vi "DoNanoCmd.vi"(4 "Relay Control Port":u32, 5 "Sense Resistor":dbl, 6 "Current Limit":dbl, 7 "Pin 2":u32, 8 "error in (no error)":errorcluster, 9 "Pin 1":u32, 10 "Nano Op":T1=enum."Get analog pin voltage", 11 "VISA resource name":refnum<visa-resource-name>="COM21") -> (0 "error out":errorcluster={"status"=FALSE, "code"=1073676294, "source"="VISA Read in DoNanoCmd.vi"}, 1 "Response length":i32, 2 "Read Value":dbl, 3 "VISA resource name 2":refnum<visa-resource-name>="COM20")   [LabVIEW 2013]
uses:
  NanoCmds.ctl
  Test Globals/Global 1.vi
panel:
  in  "SerialNotOpen? (f)":bool
  out "return count":u32
  out "timeout":bool
  in  "WaitForResponse":string
  out "read buffer":string
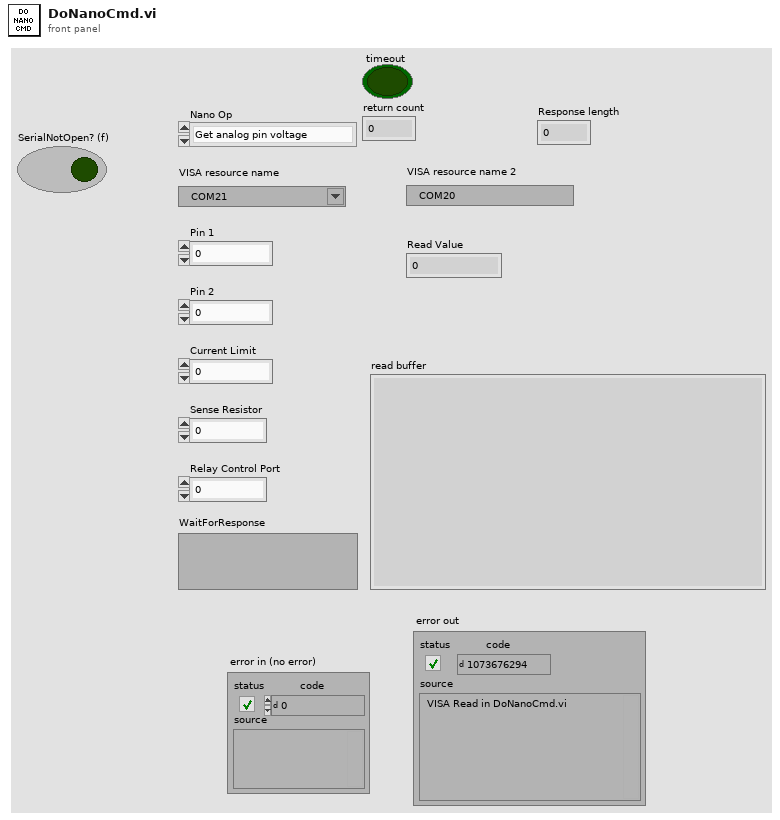
[diagram p1: front panel]
types:
  T1 = typedef "NanoCmds.ctl" = enum16{"Make digital port an output", "Make digital port an input", "Set digital pin high", "Set digital pin low", "Get digital pin state", "Get analog pin voltage", "Get analog pins difference", "Get ohms at analog pin", "Turn on current limit", "Reset Nano device", "Get digital pin state pullup", "Read current", "Initialize", "Power up uut", "Power down uut", "Get uut current draw", "Set ADC volts high", "Set ADC volts low", "Start up uut modem", "Get CTS state", "Get on_nsleep state", "Reset modem", "Get lid state", "Wait for lid closed", "Wait for lid open", "Power up, start, get curr", "Check if X2 shorted", "Power up and start up", "Check X3 shorted", "Get RTS state", "Get DTR state", "Reboot 1002759"}
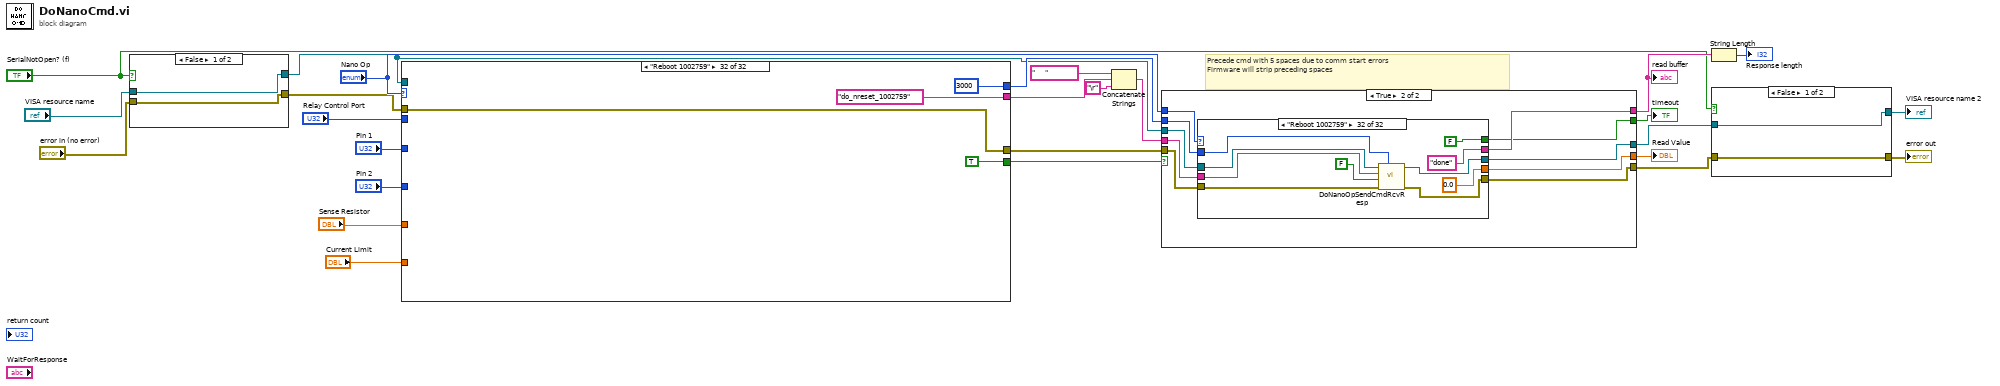
[diagram p0: block diagram]
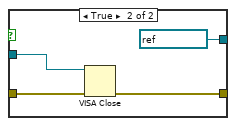
[diagram p2: hidden frame]
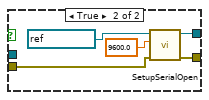
[diagram p3: hidden frame]
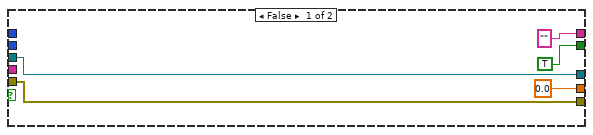
[diagram p4: hidden frame]
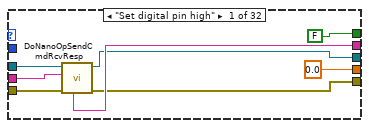
[diagram p5: hidden frame]
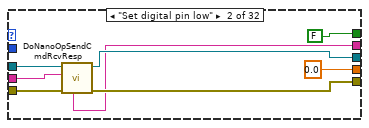
[diagram p6: hidden frame]
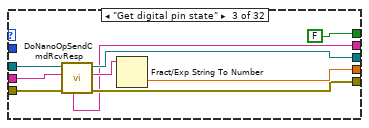
[diagram p7: hidden frame]
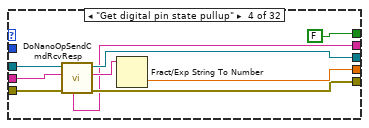
[diagram p8: hidden frame]
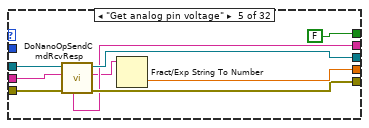
[diagram p9: hidden frame]
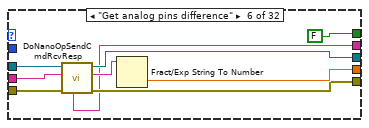
[diagram p10: hidden frame]
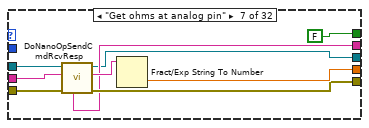
[diagram p11: hidden frame]
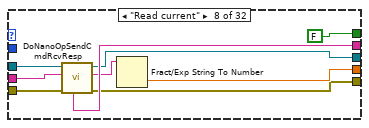
[diagram p12: hidden frame]
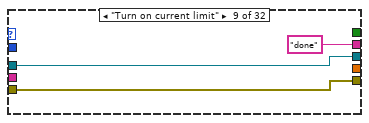
[diagram p13: hidden frame]
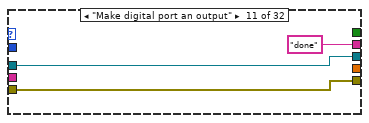
[diagram p15: hidden frame]
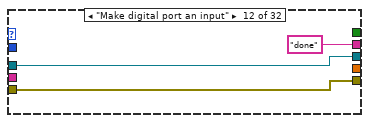
[diagram p16: hidden frame]
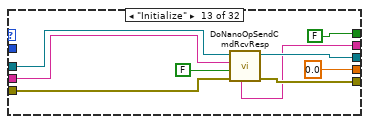
[diagram p17: hidden frame]
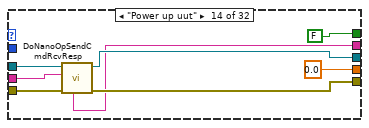
[diagram p18: hidden frame]
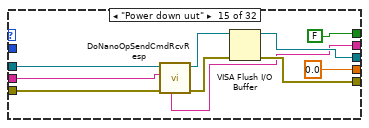
[diagram p19: hidden frame]
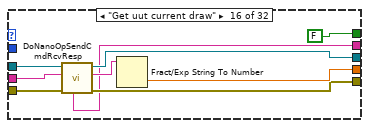
[diagram p20: hidden frame]
diagram:
  # "Precede cmd with 5 spaces due to comm start errors\nFirmware will strip preceding spaces"
  n1 = case shown="False" "SerialNotOpen? (f)" {
    tunnel: [w27 w30] -> w1
    tunnel: "error in (no error)" -> [w28 w33]
    tunnel: [w28 w29] -> w9
    tunnel: "VISA resource name" -> [w27 _]
    frame False {
    }
    frame True {
      n2 = call "SetupSerialOpen.vi"("error in (no error)"=w33, "Baud"=9600.0, "VISA Refnum in"=refnum<visa-resource-name> "COM21") -> ("error out"=w29:errorcluster, "VISA session"=w30:refnum<visa-resource-name>)  [unwired: 7 in]
    }
  }
  n3 = case shown="\"Reboot 1002759\"" "Nano Op" {
    tunnel: w9 -> [w40 w51 w55 w75 w93 w111 w126 w137 w152 _ w180 _ _ w188 w192 w196 w200 w204 w208 w212 w216 w220 w224 w227 w231 w249 w265 w268 w272 w276 w279 w284]
    tunnel: [w40 w51 w54 w74 w92 w110 w126 w137 w152 _ w182 _ _ w188 w192 w196 w200 w204 w208 w212 w216 w220 w224 w227 w231 w249 w265 w268 w272 w276 w279 w284] -> w16
    tunnel: "Pin 1" -> [w38 _ w58 w76 w94 w112 w131 w138 w153 w171 _ _ _ _ _ _ _ _ _ _ _ _ _ _ _ _ _ _ _ _ _ _]
    tunnel: [w41 "INIT" w61 w79 w97 w115 w130 w141 w156 w173 _ _ _ "power_up" "power_down" "curr" "adc_high" "adc_low" "start_up" "cts" "on_nsleep" "do_nreset" "lid" "WAITLIDCLOSED" "WAITLIDOPEN" w250 w257 "x2_shorted" "x3_shorted" "read_rts" "read_dtr" "do_nreset_1002759"] -> w19
    tunnel: "Pin 2" -> [_ _ _ _ _ _ w128 _ _ w170 _ _ _ _ _ _ _ _ _ _ _ _ _ _ _ _ _ _ _ _ _ _]
    tunnel: "Relay Control Port" -> [_ _ _ _ _ _ _ _ _ w172 _ _ _ _ _ _ _ _ _ _ _ _ _ _ _ _ _ _ _ _ _ _]
    tunnel: "Sense Resistor" -> [_ _ _ _ _ _ _ _ _ w167 _ _ _ _ _ _ _ _ _ _ _ _ _ _ _ _ _ _ _ _ _ _]
    tunnel: "Current Limit" -> [_ _ _ _ _ _ _ _ _ w166 _ _ _ _ _ _ _ _ _ _ _ _ _ _ _ _ _ _ _ _ _ _]
    tunnel: [w35 _ w56 w72 w90 w108 _ w135 w150 _ _ _ _ TRUE TRUE TRUE TRUE TRUE TRUE TRUE TRUE TRUE TRUE TRUE TRUE TRUE TRUE TRUE TRUE TRUE TRUE TRUE] -> w14
    tunnel: [u32 3000 u32 3000 u32 3000 u32 3000 u32 3000 u32 3000 u32 3000 u32 3000 u32 3000 u32 3000 u32 3000 u32 3000 u32 3000 u32 9000 u32 3000 u32 3000 u32 3000 u32 3000 u32 3000 u32 3000 u32 3000 u32 3000 u32 3000 u32 3000 u32 3000 w233 w261 u32 3000 u32 3000 u32 3000 u32 3000 u32 3000] -> w3
    tunnel: w1 -> [_ _ _ _ _ _ _ _ _ _ _ _ _ _ _ _ _ _ _ _ _ _ _ _ _ _ _ _ _ _ _ _]
    frame "Set digital pin high" {
      n4 = In Range and Coerce(upper limit=u32 13, x=w38, lower limit=u32 2) -> (In Range?=w39:bool)  [unwired: 1 out]
      n5 = case shown="True" w39 {
        selector: w39 -> [w43 w44]
        tunnel: w38 -> [_ w46]
        tunnel: ["" w45] -> w41
        tunnel: [w43 w44] -> w35
        frame False {
        }
        frame True {
          n6 = Number To Decimal String(number=w46) -> (decimal integer string=w47:string)  [unwired: 1 in]
          n7 = Concatenate Strings("DIG_HI", "," ("string"), w47) -> (w45:string)
        }
      }
    }
    frame "Initialize" {
    }
    frame "Set digital pin low" {
      n8 = In Range and Coerce(upper limit=u32 13, x=w58, lower limit=u32 2) -> (In Range?=w57:bool)  [unwired: 1 out]
      n9 = case shown="True" w57 {
        selector: w57 -> [w63 w65]
        tunnel: [_ w67] -> w61
        tunnel: w58 -> [_ w66]
        tunnel: [w63 w65] -> w56
        tunnel: w55 -> [w62 w64]
        tunnel: [w62 w64] -> w54
        frame False {
        }
        frame True {
          n10 = Number To Decimal String(number=w66) -> (decimal integer string=w68:string)  [unwired: 1 in]
          n11 = Concatenate Strings("DIG_LO", "," ("string"), w68) -> (w67:string)
        }
      }
    }
    frame "Get digital pin state" {
      n12 = In Range and Coerce(upper limit=u32 13, x=w76, lower limit=u32 2) -> (In Range?=w73:bool)  [unwired: 1 out]
      n13 = case shown="True" w73 {
        selector: w73 -> [w81 w82]
        tunnel: [_ w85] -> w79
        tunnel: w76 -> [_ w84]
        tunnel: w75 -> [w80 w83]
        tunnel: [w80 w83] -> w74
        tunnel: [w81 w82] -> w72
        frame False {
        }
        frame True {
          n14 = Number To Decimal String(number=w84) -> (decimal integer string=w86:string)  [unwired: 1 in]
          n15 = Concatenate Strings("DIG_STATE", "," ("string"), w86) -> (w85:string)
        }
      }
    }
    frame "Get digital pin state pullup" {
      n16 = In Range and Coerce(upper limit=u32 13, x=w94, lower limit=u32 2) -> (In Range?=w91:bool)  [unwired: 1 out]
      n17 = case shown="True" w91 {
        selector: w91 -> [w99 w101]
        tunnel: [_ w100] -> w97
        tunnel: w94 -> [_ w103]
        tunnel: w93 -> [w98 w102]
        tunnel: [w98 w102] -> w92
        tunnel: [w99 w101] -> w90
        frame False {
        }
        frame True {
          n18 = Number To Decimal String(number=w103) -> (decimal integer string=w104:string)  [unwired: 1 in]
          n19 = Concatenate Strings("DIG_STATE_PULLUP", "," ("string"), w104) -> (w100:string)
        }
      }
    }
    frame "Get analog pin voltage" {
      n20 = In Range and Coerce(upper limit=u32 5, x=w112, lower limit=u32 0) -> (In Range?=w109:bool)  [unwired: 1 out]
      n21 = case shown="True" w109 {
        selector: w109 -> [w117 w118]
        tunnel: [_ w121] -> w115
        tunnel: w112 -> [_ w120]
        tunnel: w111 -> [w116 w119]
        tunnel: [w116 w119] -> w110
        tunnel: [w117 w118] -> w108
        frame False {
        }
        frame True {
          n22 = Number To Decimal String(number=w120) -> (decimal integer string=w122:string)  [unwired: 1 in]
          n23 = Concatenate Strings("ANA_READ", "," ("string"), w122) -> (w121:string)
        }
      }
    }
    frame "Get analog pins difference" {
      w129 = "," ("string")
      n24 = Number To Decimal String(number=w131) -> (decimal integer string=w132:string)  [unwired: 1 in]
      n25 = Number To Decimal String(number=w128) -> (decimal integer string=w127:string)  [unwired: 1 in]
      n26 = Concatenate Strings("ANA_DIF", w129, w132, w129, w127) -> (w130:string)
    }
    frame "Get ohms at analog pin" {
      n27 = In Range and Coerce(upper limit=u32 5, x=w138, lower limit=u32 0) -> (In Range?=w136:bool)  [unwired: 1 out]
      n28 = case shown="True" w136 {
        selector: w136 -> [w142 w143]
        tunnel: [_ w145] -> w141
        tunnel: w138 -> [_ w144]
        tunnel: [w142 w143] -> w135
        frame False {
        }
        frame True {
          n29 = Number To Decimal String(number=w144) -> (decimal integer string=w146:string)  [unwired: 1 in]
          n30 = Concatenate Strings("GET_OHMS", "," ("string"), w146) -> (w145:string)
        }
      }
    }
    frame "Read current" {
      n31 = In Range and Coerce(upper limit=u32 5, x=w153, lower limit=u32 0) -> (In Range?=w151:bool)  [unwired: 1 out]
      n32 = case shown="True" w151 {
        selector: w151 -> [w157 w158]
        tunnel: [_ w160] -> w156
        tunnel: w153 -> [_ w159]
        tunnel: [w157 w158] -> w150
        frame False {
        }
        frame True {
          n33 = Number To Decimal String(number=w159) -> (decimal integer string=w161:string)  [unwired: 1 in]
          n34 = Concatenate Strings("READ_CURR", "," ("string"), w161) -> (w160:string)
        }
      }
    }
    frame "Turn on current limit" {
      w165 = i16 3 ("precision (6)")
      w174 = "," ("string")
      n35 = Number To Fractional String(number=w167, precision (6)=w165) -> (F-format string=w169:string)  [unwired: 2 in]
      n36 = Number To Fractional String(number=w166, precision (6)=w165) -> (F-format string=w168:string)  [unwired: 2 in]
      n37 = Number To Decimal String(number=w172) -> (decimal integer string=w177:string)  [unwired: 1 in]
      n38 = Number To Decimal String(number=w171) -> (decimal integer string=w176:string)  [unwired: 1 in]
      n39 = Number To Decimal String(number=w170) -> (decimal integer string=w175:string)  [unwired: 1 in]
      n40 = Concatenate Strings("CURR_LIMIT", w174, w177, w174, w176, w174, w175, w174, w169, w174, w168) -> (w173:string)
    }
    frame "Reset Nano device" {
      n41 = call "WaitMsecs.vi"("error in (no error)"=w180, "Wait Msecs"=1500.0) -> ("error out"=w182:errorcluster)  [unwired: 9 in]
    }
    frame "Make digital port an output" {
    }
    frame "Make digital port an input" {
    }
    frame "Power up uut" {
    }
    frame "Power down uut" {
    }
    frame "Get uut current draw" {
    }
    frame "Set ADC volts high" {
    }
    frame "Set ADC volts low" {
    }
    frame "Start up uut modem" {
    }
    frame "Get CTS state" {
    }
    frame "Get on_nsleep state" {
    }
    frame "Reset modem" {
    }
    frame "Get lid state" {
    }
    frame "Wait for lid closed" {
    }
    frame "Wait for lid open" {
    }
    frame "Power up, start, get curr" {
      # "calc timeout"
      n42 = global read "Global 1.vi" "Modem Make"() -> (w242:string)
      n43 = Equal?(x=w242, y="wnc") -> (x = y?=w240:bool)
      n44 = Equal?(x=w242, y="sequans") -> (x = y?=w241:bool)
      n45 = Or(x=w240, y=w241) -> (x .or. y?=w239:bool)
      n46 = global read "Global 1.vi" "reset delay"() -> (w236:u32)
      n47 = Select(t=3000, s=w239, f=3000) -> (s? t:f=w235:i32)
      n48 = Select(t=",9999" ("string"), s=w239, f=",3000" ("string")) -> (s? t:f=w244:string)
      n49 = Number To Decimal String(number=w236) -> (decimal integer string=w251:string)  [unwired: 1 in]
      n50 = Concatenate Strings("pstart_getcurr," ("string"), w251, w244) -> (w250:string)
      n51 = Compound Arithmetic op=ADD(w236, w235, 3000 ("value")) -> (w233:u32)
    }
    frame "Power up and start up" {
      # "calc timeout"
      n52 = global read "Global 1.vi" "on_off_wait"() -> (w260:u32)
      n53 = global read "Global 1.vi" "reset delay"() -> (w263:u32)
      n54 = Number To Decimal String(number=w263) -> (decimal integer string=w256:string)  [unwired: 1 in]
      n55 = Number To Decimal String(number=w260) -> (decimal integer string=w254:string)  [unwired: 1 in]
      n56 = call <vilib>:"Trim Whitespace.vi"("string"=w256) -> ("trimmed string"=w255:string)  [unwired: 1 in]
      n57 = call <vilib>:"Trim Whitespace.vi"("string"=w254) -> ("trimmed string"=w253:string)  [unwired: 1 in]
      n58 = Concatenate Strings("pu," ("string"), w255, "," ("string"), w253) -> (w257:string)
      n59 = Compound Arithmetic op=ADD(w263, 3000, 3000 ("value")) -> (w261:u32)
    }
    frame "Check if X2 shorted" {
    }
    frame "Check X3 shorted" {
    }
    frame "Get RTS state" {
    }
    frame "Get DTR state" {
    }
    frame "Reboot 1002759" {
    }
  }
  n60 = Concatenate Strings("     " ("string"), w19, "\r") -> (w17:string)
  n61 = case shown="True" w14 {
    tunnel: "Nano Op" -> [_ w301]
    tunnel: [0.0 w300] -> w20
    tunnel: w17 -> [_ w299]
    tunnel: w16 -> [w290 w298]
    tunnel: ["" ("read buffer") w297] -> w12
    tunnel: [TRUE ("timeout") w296] -> w15
    tunnel: [w290 w295] -> w7
    tunnel: w1 -> [w291 w294]
    tunnel: [w291 w293] -> w6
    tunnel: w3 -> [_ w292]
    frame False {
    }
    frame True {
      n62 = case shown="\"Reboot 1002759\"" w301 {
        tunnel: w294 -> [w306 w314 w322 w331 w340 w349 w358 w367 w374 w376 w380 w383 w388 w397 w405 w415 w424 w434 w442 w451 w460 w471 w479 w488 w496 w505 w517 w529 w541 w552 w560 w570]
        tunnel: w298 -> [w307 w316 w324 w333 w342 w351 w360 w369 w373 w377 w379 w382 w390 w399 w407 w417 w426 w436 w444 w453 w462 w472 w481 w490 w498 w507 w518 w531 w543 w551 w562 w572]
        tunnel: [w303 w312 w319 w329 w338 w348 w357 w365 w373 w377 w379 w382 w387 w395 w409 w413 w422 w432 w440 w449 w458 w468 w477 w487 w494 w502 w515 w530 w542 w546 w557 w568] -> w295
        tunnel: [0.0 0.0 w326 w335 w344 w353 w362 w371 _ _ _ _ 0.0 0.0 0.0 w419 0.0 0.0 0.0 w455 w464 0.0 ("f") w483 0.0 0.0 w509 0.0 ("f") w520 w532 w547 w556 0.0 ("f")] -> w300
        tunnel: w299 -> [w305 w315 w323 w332 w341 w350 w359 w368 _ w375 _ _ w389 w398 w406 w416 w425 w435 w443 w452 w461 w469 w480 w489 w497 w506 w510 w528 w540 w550 w559 w571]
        tunnel: [w304 w310 w318 w327 w337 w345 w355 w366 "done" ("read buffer") w375 "done" ("read buffer") "done" ("read buffer") w385 w394 w401 w411 w421 w431 w439 w446 w456 "done" ("read buffer") w476 w484 w492 w501 w514 w526 w538 w545 w558 "done" ("read buffer")] -> w297
        tunnel: [FALSE ("timeout") FALSE ("timeout") FALSE ("timeout") FALSE ("timeout") FALSE ("timeout") FALSE ("timeout") FALSE ("timeout") FALSE ("timeout") _ _ _ _ FALSE ("timeout") FALSE ("timeout") FALSE ("timeout") FALSE ("timeout") FALSE ("timeout") FALSE ("timeout") FALSE ("timeout") FALSE ("timeout") FALSE ("timeout") FALSE ("timeout") FALSE ("timeout") FALSE ("timeout") FALSE ("timeout") FALSE ("timeout") FALSE ("timeout") FALSE ("timeout") FALSE ("timeout") FALSE ("timeout") FALSE ("timeout") FALSE ("timeout")] -> w296
        tunnel: [w302 w311 w321 w328 w339 w347 w354 w363 w374 w376 w380 w383 w386 w396 w410 w414 w423 w433 w441 w450 w459 w470 w478 w486 w495 w503 w516 w527 w539 w548 w555 w565] -> w293
        tunnel: w292 -> [_ _ _ _ _ _ _ _ _ _ _ _ _ _ _ _ _ _ _ w447 _ w466 _ _ _ w500 w513 _ _ w544 w561 w569]
        frame "Set digital pin high" {
          n63 = call "DoNanoOpSendCmdRcvResp.vi"("error in (no error)"=w307, "Cmd String"=w305, "VISA resource name"=w306) -> ("error out"=w303:errorcluster, "VISA resource name out"=w302:refnum<visa-resource-name>, "read buffer"=w304:string)  [unwired: 2 in, 4 out]
        }
        frame "Set digital pin low" {
          n64 = call "DoNanoOpSendCmdRcvResp.vi"("error in (no error)"=w316, "Cmd String"=w315, "VISA resource name"=w314) -> ("error out"=w312:errorcluster, "VISA resource name out"=w311:refnum<visa-resource-name>, "read buffer"=w310:string)  [unwired: 2 in, 4 out]
        }
        frame "Get digital pin state" {
          n65 = call "DoNanoOpSendCmdRcvResp.vi"("error in (no error)"=w324, "Cmd String"=w323, "VISA resource name"=w322) -> ("error out"=w319:errorcluster, "Line 1"=w320:string, "VISA resource name out"=w321:refnum<visa-resource-name>, "read buffer"=w318:string)  [unwired: 2 in, 3 out]
          n66 = Fract/Exp String To Number(string=w320) -> (number=w326:dbl)  [unwired: 3 in, 1 out]
        }
        frame "Get digital pin state pullup" {
          n67 = call "DoNanoOpSendCmdRcvResp.vi"("error in (no error)"=w333, "Cmd String"=w332, "VISA resource name"=w331) -> ("error out"=w329:errorcluster, "Line 1"=w330:string, "VISA resource name out"=w328:refnum<visa-resource-name>, "read buffer"=w327:string)  [unwired: 2 in, 3 out]
          n68 = Fract/Exp String To Number(string=w330) -> (number=w335:dbl)  [unwired: 3 in, 1 out]
        }
        frame "Get analog pin voltage" {
          n69 = call "DoNanoOpSendCmdRcvResp.vi"("error in (no error)"=w342, "Cmd String"=w341, "VISA resource name"=w340) -> ("error out"=w338:errorcluster, "Line 1"=w336:string, "VISA resource name out"=w339:refnum<visa-resource-name>, "read buffer"=w337:string)  [unwired: 2 in, 3 out]
          n70 = Fract/Exp String To Number(string=w336) -> (number=w344:dbl)  [unwired: 3 in, 1 out]
        }
        frame "Get analog pins difference" {
          n71 = call "DoNanoOpSendCmdRcvResp.vi"("error in (no error)"=w351, "Cmd String"=w350, "VISA resource name"=w349) -> ("error out"=w348:errorcluster, "Line 1"=w346:string, "VISA resource name out"=w347:refnum<visa-resource-name>, "read buffer"=w345:string)  [unwired: 2 in, 3 out]
          n72 = Fract/Exp String To Number(string=w346) -> (number=w353:dbl)  [unwired: 3 in, 1 out]
        }
        frame "Get ohms at analog pin" {
          n73 = call "DoNanoOpSendCmdRcvResp.vi"("error in (no error)"=w360, "Cmd String"=w359, "VISA resource name"=w358) -> ("error out"=w357:errorcluster, "Line 1"=w356:string, "VISA resource name out"=w354:refnum<visa-resource-name>, "read buffer"=w355:string)  [unwired: 2 in, 3 out]
          n74 = Fract/Exp String To Number(string=w356) -> (number=w362:dbl)  [unwired: 3 in, 1 out]
        }
        frame "Read current" {
          n75 = call "DoNanoOpSendCmdRcvResp.vi"("error in (no error)"=w369, "Cmd String"=w368, "VISA resource name"=w367) -> ("error out"=w365:errorcluster, "Line 1"=w364:string, "VISA resource name out"=w363:refnum<visa-resource-name>, "read buffer"=w366:string)  [unwired: 2 in, 3 out]
          n76 = Fract/Exp String To Number(string=w364) -> (number=w371:dbl)  [unwired: 3 in, 1 out]
        }
        frame "Turn on current limit" {
        }
        frame "Reset Nano device" {
        }
        frame "Make digital port an output" {
        }
        frame "Make digital port an input" {
        }
        frame "Initialize" {
          n77 = call "DoNanoOpSendCmdRcvResp.vi"("error in (no error)"=w390, "Wait after response"=FALSE, "Cmd String"=w389, "VISA resource name"=w388) -> ("error out"=w387:errorcluster, "VISA resource name out"=w386:refnum<visa-resource-name>, "read buffer"=w385:string)  [unwired: 1 in, 4 out]
        }
        frame "Power up uut" {
          n78 = call "DoNanoOpSendCmdRcvResp.vi"("error in (no error)"=w399, "Cmd String"=w398, "VISA resource name"=w397) -> ("error out"=w395:errorcluster, "VISA resource name out"=w396:refnum<visa-resource-name>, "read buffer"=w394:string)  [unwired: 2 in, 4 out]
        }
        frame "Power down uut" {
          n79 = call "DoNanoOpSendCmdRcvResp.vi"("error in (no error)"=w407, "Cmd String"=w406, "VISA resource name"=w405) -> ("error out"=w402:errorcluster, "VISA resource name out"=w404:refnum<visa-resource-name>, "read buffer"=w401:string)  [unwired: 2 in, 4 out]
          n80 = VISA Flush I/O Buffer(VISA resource name=w404, error in (no error)=w402) -> (VISA resource name out=w410:refnum<visa-resource-name>, error out=w409:errorcluster)  [unwired: 1 in]
        }
        frame "Get uut current draw" {
          n81 = call "DoNanoOpSendCmdRcvResp.vi"("error in (no error)"=w417, "Cmd String"=w416, "VISA resource name"=w415) -> ("error out"=w413:errorcluster, "Line 1"=w412:string, "VISA resource name out"=w414:refnum<visa-resource-name>, "read buffer"=w411:string)  [unwired: 2 in, 3 out]
          n82 = Fract/Exp String To Number(string=w412) -> (number=w419:dbl)  [unwired: 3 in, 1 out]
        }
        frame "Set ADC volts high" {
          n83 = call "DoNanoOpSendCmdRcvResp.vi"("error in (no error)"=w426, "Wait after response"=FALSE, "Cmd String"=w425, "VISA resource name"=w424) -> ("error out"=w422:errorcluster, "VISA resource name out"=w423:refnum<visa-resource-name>, "read buffer"=w421:string)  [unwired: 1 in, 4 out]
        }
        frame "Set ADC volts low" {
          n84 = call "DoNanoOpSendCmdRcvResp.vi"("error in (no error)"=w436, "Wait after response"=FALSE, "Cmd String"=w435, "VISA resource name"=w434) -> ("error out"=w432:errorcluster, "VISA resource name out"=w433:refnum<visa-resource-name>, "read buffer"=w431:string)  [unwired: 1 in, 4 out]
        }
        frame "Start up uut modem" {
          n85 = call "DoNanoOpSendCmdRcvResp.vi"("error in (no error)"=w444, "Cmd String"=w443, "VISA resource name"=w442) -> ("error out"=w440:errorcluster, "VISA resource name out"=w441:refnum<visa-resource-name>, "read buffer"=w439:string)  [unwired: 2 in, 4 out]
        }
        frame "Get CTS state" {
          n86 = call "DoNanoOpSendCmdRcvResp.vi"("Expected response time (msecs)"=w447, "error in (no error)"=w453, "Cmd String"=w452, "VISA resource name"=w451) -> ("error out"=w449:errorcluster, "Line 1"=w448:string, "VISA resource name out"=w450:refnum<visa-resource-name>, "read buffer"=w446:string)  [unwired: 1 in, 3 out]
          n87 = Fract/Exp String To Number(string=w448) -> (number=w455:dbl)  [unwired: 3 in, 1 out]
        }
        frame "Get on_nsleep state" {
          n88 = call "DoNanoOpSendCmdRcvResp.vi"("error in (no error)"=w462, "Cmd String"=w461, "VISA resource name"=w460) -> ("error out"=w458:errorcluster, "Line 1"=w457:string, "VISA resource name out"=w459:refnum<visa-resource-name>, "read buffer"=w456:string)  [unwired: 2 in, 3 out]
          n89 = Fract/Exp String To Number(string=w457) -> (number=w464:dbl)  [unwired: 3 in, 1 out]
        }
        frame "Reset modem" {
          n90 = call "DoNanoOpSendCmdRcvResp.vi"("Expected response time (msecs)"=w466, "error in (no error)"=w472, "Wait after response"=FALSE, "Cmd String"=w469, "VISA resource name"=w471) -> ("error out"=w468:errorcluster, "VISA resource name out"=w470:refnum<visa-resource-name>)  [unwired: 5 out]
        }
        frame "Get lid state" {
          n91 = call "DoNanoOpSendCmdRcvResp.vi"("error in (no error)"=w481, "Cmd String"=w480, "VISA resource name"=w479) -> ("error out"=w477:errorcluster, "Line 1"=w475:string, "VISA resource name out"=w478:refnum<visa-resource-name>, "read buffer"=w476:string)  [unwired: 2 in, 3 out]
          n92 = Fract/Exp String To Number(string=w475) -> (number=w483:dbl)  [unwired: 3 in, 1 out]
        }
        frame "Wait for lid closed" {
          n93 = call "DoNanoOpSendCmdRcvResp.vi"("error in (no error)"=w490, "Cmd String"=w489, "VISA resource name"=w488) -> ("error out"=w487:errorcluster, "VISA resource name out"=w486:refnum<visa-resource-name>, "read buffer"=w484:string)  [unwired: 2 in, 4 out]
        }
        frame "Wait for lid open" {
          n94 = call "DoNanoOpSendCmdRcvResp.vi"("error in (no error)"=w498, "Cmd String"=w497, "VISA resource name"=w496) -> ("error out"=w494:errorcluster, "VISA resource name out"=w495:refnum<visa-resource-name>, "read buffer"=w492:string)  [unwired: 2 in, 4 out]
        }
        frame "Power up, start, get curr" {
          n95 = call "DoNanoOpSendCmdRcvResp.vi"("Expected response time (msecs)"=w500, "error in (no error)"=w507, "Cmd String"=w506, "VISA resource name"=w505) -> ("error out"=w502:errorcluster, "Line 1"=w504:string, "VISA resource name out"=w503:refnum<visa-resource-name>, "read buffer"=w501:string)  [unwired: 1 in, 3 out]
          n96 = Fract/Exp String To Number(string=w504) -> (number=w509:dbl)  [unwired: 3 in, 1 out]
        }
        frame "Power up and start up" {
          n97 = call "DoNanoOpSendCmdRcvResp.vi"("Expected response time (msecs)"=w513, "error in (no error)"=w518, "Wait after response"=TRUE, "Cmd String"=w510, "VISA resource name"=w517) -> ("error out"=w515:errorcluster, "VISA resource name out"=w516:refnum<visa-resource-name>, "read buffer"=w514:string)  [unwired: 4 out]
        }
        frame "Check if X2 shorted" {
          n98 = call "DoNanoOpSendCmdRcvResp.vi"("error in (no error)"=w531, "Cmd String"=w528, "VISA resource name"=w529) -> ("error out"=w530:errorcluster, "Line 1"=w526:string, "VISA resource name out"=w527:refnum<visa-resource-name>)  [unwired: 2 in, 4 out]
          n99 = Equal?(x=w526, y="YES") -> (x = y?=w523:bool)
          n100 = Select(t=1.0, s=w523, f=0.0) -> (s? t:f=w520:dbl)
        }
        frame "Check X3 shorted" {
          n101 = call "DoNanoOpSendCmdRcvResp.vi"("error in (no error)"=w543, "Cmd String"=w540, "VISA resource name"=w541) -> ("error out"=w542:errorcluster, "Line 1"=w538:string, "VISA resource name out"=w539:refnum<visa-resource-name>)  [unwired: 2 in, 4 out]
          n102 = Equal?(x=w538, y="YES") -> (x = y?=w535:bool)
          n103 = Select(t=1.0, s=w535, f=0.0) -> (s? t:f=w532:dbl)
        }
        frame "Get RTS state" {
          n104 = call "DoNanoOpSendCmdRcvResp.vi"("Expected response time (msecs)"=w544, "error in (no error)"=w551, "Cmd String"=w550, "VISA resource name"=w552) -> ("error out"=w546:errorcluster, "Line 1"=w553:string, "VISA resource name out"=w548:refnum<visa-resource-name>, "read buffer"=w545:string)  [unwired: 1 in, 3 out]
          n105 = Fract/Exp String To Number(string=w553) -> (number=w547:dbl)  [unwired: 3 in, 1 out]
        }
        frame "Get DTR state" {
          n106 = call "DoNanoOpSendCmdRcvResp.vi"("Expected response time (msecs)"=w561, "error in (no error)"=w562, "Cmd String"=w559, "VISA resource name"=w560) -> ("error out"=w557:errorcluster, "Line 1"=w563:string, "VISA resource name out"=w555:refnum<visa-resource-name>, "read buffer"=w558:string)  [unwired: 1 in, 3 out]
          n107 = Fract/Exp String To Number(string=w563) -> (number=w556:dbl)  [unwired: 3 in, 1 out]
        }
        frame "Reboot 1002759" {
          n108 = call "DoNanoOpSendCmdRcvResp.vi"("Expected response time (msecs)"=w569, "error in (no error)"=w572, "Wait after response"=FALSE, "Cmd String"=w571, "VISA resource name"=w570) -> ("error out"=w568:errorcluster, "VISA resource name out"=w565:refnum<visa-resource-name>)  [unwired: 5 out]
        }
      }
    }
  }
  "Read Value" <- w20
  "read buffer" <- w12
  "timeout" <- w15
  n109 = String Length(string=w12) -> (length=→"Response length":i32)
  n110 = case shown="False" "SerialNotOpen? (f)" {
    tunnel: [w575 w578] -> w8
    tunnel: w7 -> [w575 w579]
    tunnel: w6 -> [w574 w577]
    tunnel: [w574 refnum<visa-resource-name> "COM21" ("VISA resource name out")] -> w5
    frame False {
    }
    frame True {
      n111 = VISA Close(VISA resource name=w577, error in (no error)=w579) -> (error out=w578:errorcluster)
    }
  }
  "error out" <- w8
  "VISA resource name 2" <- w5
